vi "Mono_init.vi"(8 "error in (no error)":errorcluster) -> (0 "error out":errorcluster, 1 "Mono Connected?":bool, 3 "CmdLib":refnum<k24>)   [LabVIEW 2017]
uses:
  C:/Users/Admin/Desktop/connection test/Cornerstone.dll
  Cornerstone.dll
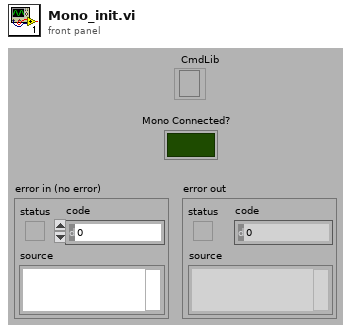
[diagram p1: front panel]
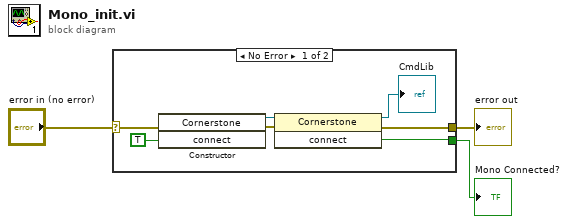
[diagram p0: block diagram]
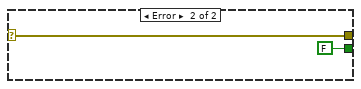
[diagram p2: hidden frame]
diagram:
  n1 = case shown="No Error" "error in (no error)" {
    selector: "error in (no error)" -> [w10 w12]
    tunnel: [w5 w12] -> w2
    tunnel: [w6 FALSE] -> w1
    frame No Error {
      n2 = constructor class="Cornerstone"(error in=w10, "connect"=TRUE) -> (reference out=w8:refnum<k24>, error out=w7:errorcluster)  [unwired: 2 in, 2 out]
      n3 = invoke class="Cornerstone" method="connect"(reference=w8, error in=w7) -> (reference out=→"CmdLib":refnum<k24>, error out=w5:errorcluster, "connect"=w6:bool)  [unwired: 1 in]
    }
    frame Error {
    }
  }
  "error out" <- w2
  "Mono Connected?" <- w1
